vi "Read MonoPubSubData.vi"(8 "error in (no error)":errorcluster, 11 "Monochromator in":refnum<class "Monochromator.lvclass">) -> (0 "error out":errorcluster, 2 "MonoPubSubData.lvclass":refnum<class "MonoPubSubData.lvclass">, 3 "Monochromator out":refnum<class "Monochromator.lvclass">)   [LabVIEW 2016, in "Monochromator.lvclass"]
uses:
  Monochromator.lvclass
  MonoPubSubData/MonoPubSubData.lvclass
  Monochromator.lvclass/Monochromator.ctl
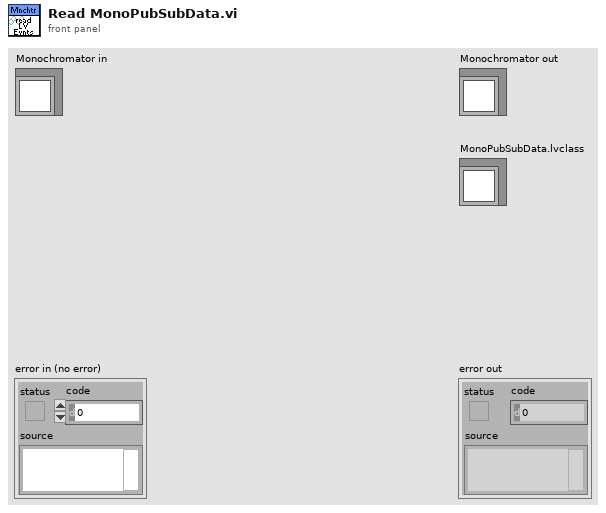
[diagram p1: front panel]
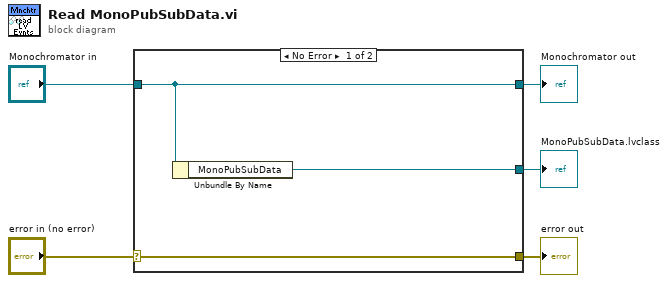
[diagram p0: block diagram]
diagram:
  n1 = case shown="No Error" "error in (no error)" {
    selector: "error in (no error)" -> [w8 w9]
    tunnel: [w8 w9] -> w4
    tunnel: [w7 w10] -> w2
    tunnel: "Monochromator in" -> [w7 w10]
    tunnel: [w6 _] -> w1
    frame No Error {
      n2 = Unbundle By Name(w7) -> ("MonoPubSubData"=w6:refnum<class "MonoPubSubData.lvclass">)
    }
    frame Error {
    }
  }
  "error out" <- w4
  "Monochromator out" <- w2
  "MonoPubSubData.lvclass" <- w1
